vi "1 IDE.vi"() -> ()   [LabVIEW 2015]
panel:
  out "Numeric Indicator":dbl
  in  "Numeric Control":dbl
  out "Gauge":dbl(knob) scale=0.0..100.0
  in  "Knob":dbl(knob) scale=0.0..100.0
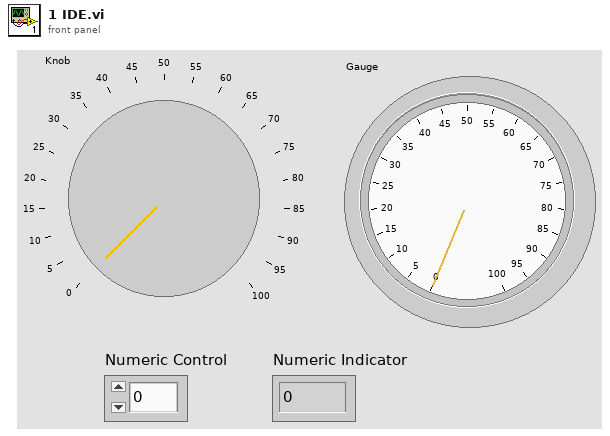
[diagram p1: front panel]
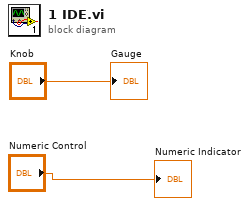
[diagram p0: block diagram]
diagram:
  "Gauge" <- "Knob"
  "Numeric Indicator" <- "Numeric Control"
